vi "Helmholtz2D_FEM_Triangulation.vi"(11 "Helmholtz2D FEM Data In":T1) -> (3 "Helmholtz2D FEM Data Out":T1)   [LabVIEW 2020, in "NI_PDE.lvlib"]
uses:
  <vilib>/gmath/NI_PDE.lvlib
  <vilib>/gmath/pde.llb/Helmholtz2D_FEM/Helmholtz2D_FEM_Data.ctl
  <vilib>/gmath/pde.llb/Common/PDE_Sparse Mtrx.ctl
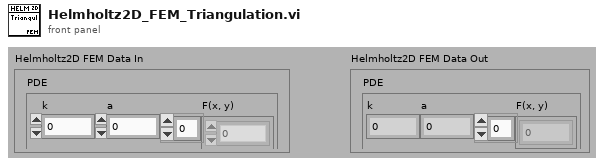
[diagram p1: front panel]
types:
  T1 = typedef "NI_PDE.lvlib/Helmholtz2D_FEM_Data.ctl" = cluster{"PDE":cluster{"k":dbl, "a":dbl, "F(x, y)":dbl[]}, "# of unknown":i32, "# of known":i32, "U(x, y)":dbl[], "X Used":dbl[], "Y Used":dbl[], "Triangulation":i32[][], "Coef Mtrx":T2}
  T2 = typedef "NI_PDE.lvlib/PDE_Sparse Mtrx.ctl" = cluster{"Row":cluster{"col":i32, "value":dbl}[]}[]
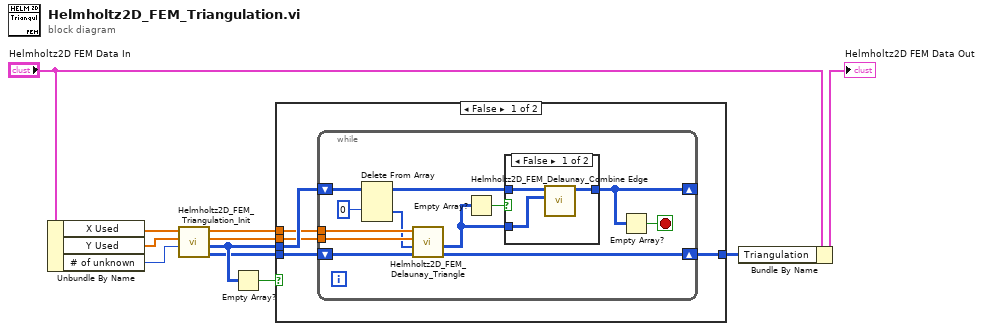
[diagram p0: block diagram]
diagram:
  n1 = Unbundle By Name("Helmholtz2D FEM Data In") -> ("X Used"=w4:dbl[], "Y Used"=w3:dbl[], "# of unknown"=w2:i32)
  n2 = call <vilib>:"Helmholtz2D_FEM_Triangulation_Init.vi"("# of unknown"=w2, "Y In"=w3, "X In"=w4) -> ("Triangulation"=w5:i32[][], "Edges"=w6:i32[][], "Y Out"=w7:dbl[], "X Out"=w8:dbl[])  [unwired: 5 out]
  n3 = Empty Array?(array=w6) -> (empty?=w9:bool)
  n4 = case shown="False" w9 {
    tunnel: w6 -> [w16 _]
    tunnel: [w15 w33] -> w1
    tunnel: w7 -> [w14 _]
    tunnel: w8 -> [w13 _]
    tunnel: w5 -> [w12 w33]
    frame False {
      n5 = while {
        shift-right: [w24] -> _
        shift-left: w16 -> [w25]
        shift-right: [w18] -> w15
        shift-left: w12 -> [w20]
        tunnel: w13 -> [w27]
        tunnel: w14 -> [w28]
        stop <- w23 stop-if-true
        n6 = Delete From Array(array=w25, index (row)=0) -> (deleted portion=w22:i32[], array with subset deleted=w26:i32[][])  [unwired: 2 in]
        n7 = call <vilib>:"Helmholtz2D_FEM_Delaunay_Triangle.vi"("Triangles In"=w20, "Index"=w22, "Y"=w28, "X"=w27) -> ("Triangles Out"=w18:i32[][], "Edges"=w19:i32[][])  [unwired: 1 in, 5 out]
        n8 = Empty Array?(array=w19) -> (empty?=w21:bool)
        n9 = case shown="False" w21 {
          tunnel: w26 -> [w31 w32]
          tunnel: [w30 w32] -> w24
          tunnel: w19 -> [w29 _]
          frame False {
            n10 = call <vilib>:"Helmholtz2D_FEM_Delaunay_Combine Edge.vi"("New Edges"=w29, "Edges in"=w31) -> ("Edges Out"=w30:i32[][])  [unwired: 9 out]
          }
          frame True {
          }
        }
        n11 = Empty Array?(array=w24) -> (empty?=w23:bool)
      }
    }
    frame True {
    }
  }
  n12 = Bundle By Name(cluster="Helmholtz2D FEM Data In", "Triangulation"=w1) -> (→"Helmholtz2D FEM Data Out":T1)
